vi "TEMPSING.VI"() -> ()   [LabVIEW 2021]
panel:
  in  "Lakeshore Address":string
  out "Temperature output":ext format="%.2f"
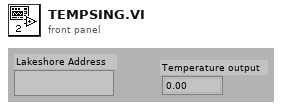
[diagram p1: front panel]
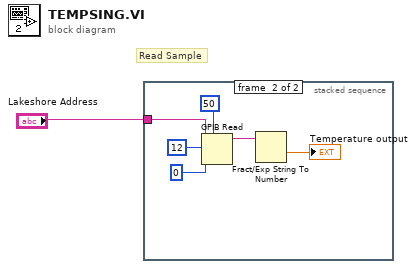
[diagram p0: block diagram]
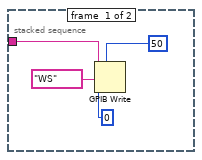
[diagram p2: hidden frame]
diagram:
  # "Read Sample"
  n1 = stacked-sequence {
    tunnel: "Lakeshore Address" -> [w2 w6]
    frame #0 {
      n2 = GPIB Write(0:w2, 1:"WS", 2:0, 4:50) -> ()  [unwired: 1 in, 2 out]
    }
    frame #1 {
      n3 = GPIB Read(0:w6, 1:12, 2:0, 4:50) -> (5:w9:string)  [unwired: 1 in, 2 out]
      n4 = Fract/Exp String To Number(string=w9) -> (number=→"Temperature output":dbl)  [unwired: 3 in, 1 out]
    }
  }
